vi "FPGA Main.vi"() -> ()   [LabVIEW 2016]
uses:
  <vilib>/Platform/TimedLoop/XDataNode/timing_clust.ctl
  <vilib>/Platform/TimedLoop/XDataNode/nitl_modes.ctl
  <vilib>/Platform/TimedLoop/XDataNode/wakeup.ctl
  <vilib>/rvi/Emulation/niFpgaGetClockAttributes.vi
  <vilib>/rvi/Emulation/niFpgaSctlEmulationGetInTimedLoop.vi
  <vilib>/rvi/Emulation/niFpgaEmulationReportErrorSimple.vi
  <vilib>/rvi/eio/common/nirviEmuTemplateMethod_errors.vi
  <vilib>/rvi/Emulation/niFpgaCriticalErrorInLSC.vi
  <vilib>/eio/EIONode/EIONode.xnode
  <vilib>/platform/TimedLoop/XDataNode/XDataNode.xnode
  <vilib>/Platform/TimedLoop/XDataNode/XDNodeRunTimeDep.lvlib
panel:
  in  "pause":bool
  in  "loop time [ms]":u32=100
  out "LEDb":bool
  out "LEDa":bool
  out "paused":bool
  # "FPGA blinker"
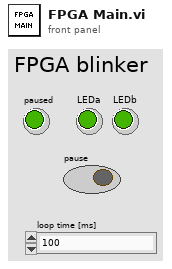
[diagram p1: front panel]
types:
  T1 = typedef "XDNodeRunTimeDep.lvlib/timing_clust.ctl" = cluster{"Expected End [f-1]":u64, "Actual End [f-1]":u64, "Finished Late? [f-1]":bool, "Expected End [i-1]":u64, "Actual End [i-1]":u64, "Finished Late? [i-1]":bool, "Expected Start [i]":u64, "Actual Start [i]":u64, "Expected Start [f]":u64, "Actual Start [f]":u64, "Source Name":string, "Structure Name":string, "Period":i64, "Deadline":i64, "Offset":i64, "Start":i64, "Priority":i32, "Timeout":i32, "Mode":T2, "Wakeup Reason":T3, "Error":errorcluster, "Source Type":string, "Secondary Source Type":string, "Global End Time":u64, "Global Start Time":u64, "Frame Duration":u64, "Iteration Duration":u64, "Assigned CPU":i32, "I/O Scan Engine Mode":u32}
  T2 = typedef "XDNodeRunTimeDep.lvlib/nitl_modes.ctl" = enum32{"No Change", "Process missed periods, maintain original phase", "Discard missed periods, maintain original phase", "Process missed periods, ignore original phase", "Discard missed periods, ignore original phase"}
  T3 = typedef "XDNodeRunTimeDep.lvlib/wakeup.ctl" = enum32{"Normal", "Aborted", "Asynchronous wakeup", "Timing source error", "Timed loop error", "Timeout"}
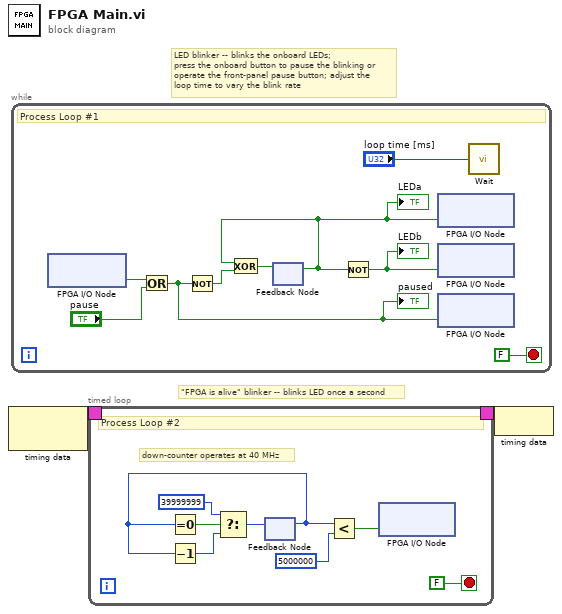
[diagram p0: block diagram]
diagram:
  # "\"FPGA is alive\" blinker -- blinks LED once a second"
  # "LED blinker -- blinks the onboard LEDs;\npress the onboard button to pause the blinking or\noperate the front-panel pause button; adjust the\nloop time to vary the blink rate"
  n1 = node-c288() -> (w2:T1)  [unwired: 1 in]
  n2 = while {
    stop <- FALSE stop-if-true
    # "Process Loop #1"
    n3 = xnode "FPGA I/O Node"() -> ("Button0"=w4:bool)  [unwired: 1 in, 1 out]
    n4 = Or(x=w4, y="pause") -> (x .or. y?=w5:bool)
    "paused" <- w5
    n5 = Not(x=w5) -> (.not. x?=w6:bool)
    n6 = feedback #1() -> (w10:bool)  [unwired: 1 in]
    "LEDa" <- w10
    n7 = Exclusive Or(1:w6, 2:w10) -> (0:w11:bool)
    n8 = feedback-in #1(w11) -> ()
    n9 = Not(x=w10) -> (.not. x?=w9:bool)
    "LEDb" <- w9
    n10 = xnode "FPGA I/O Node"("LED2"=w10) -> ()  [unwired: 1 in, 1 out]
    n11 = xnode "FPGA I/O Node"("LED3"=w9) -> ()  [unwired: 1 in, 1 out]
    n12 = xnode "FPGA I/O Node"("LED1"=w5) -> ()  [unwired: 1 in, 1 out]
    n13 = call "Wait"("Count(mSec)"="loop time [ms]") -> ()  [unwired: 1 out]
  }
  n14 = timed-loop {
    timing: w2 -> [_]
    timing-out: [_] -> w1
    stop <- FALSE stop-if-true
    # "down-counter operates at 40 MHz"
    # "Process Loop #2"
    n15 = feedback #2() -> (w14:u32)  [unwired: 1 in]
    n16 = Equal To 0?(x=w14) -> (x = 0?=w16:bool)
    n17 = Decrement(x=w14) -> (x-1=w15:u32)
    n18 = Select(t=u32 39999999, s=w16, f=w15) -> (s? t:f=w17:u32)
    n19 = feedback-in #2(w17) -> ()
    n20 = Less?(x=w14, y=u32 5000000) -> (x < y?=w12:bool)
    n21 = xnode "FPGA I/O Node"("LED0"=w12) -> ()  [unwired: 1 in, 1 out]
  }
  n22 = node-c288(w1) -> ()
